vi "joystick control bjorn.vi"() -> ()   [LabVIEW 2016, in "Aerotech VIs.lvlib"]
uses:
  Aerotech VIs.lvlib
  Motion/EnableMultiple.vi
  Motion/HomeSingle.vi
  Motion/DisableMultiple.vi
panel:
  out "Position Feedback":dbl
  in  "u home":bool
  in  "z home":bool
  in  "y home":bool
  in  "x home":bool
  out "U - Position":string
  out "Z - Position":string
  out "Y - Position":string
  out "Selection Number":u32
  in  "U control":bool
  out "u on":bool
  in  "stop":bool
  in  "Joystick On":bool
  in  "Z control":bool
  in  "Y control":bool
  in  "X control":bool
  out "z on":bool
  out "y on":bool
  out "x on":bool
  out "taskId":i32(ring) items=["TLibrary", "T01", "T02", "T03", "T04", "T05", "T06", "T07", "T08", "T09", "T10", "T11", "T12", "T13", "T14", "T15", "T16", "T17", "T18", "T19", "T20", "T21", "T22", "T23", "T24", "T25", "T26", "T27", "T28", "T29", "T30", "T31"]
  # "Do not select more than two values."
  # "Must turn off joystick before changing values. To do so press button on analog stick."
  # "Selection number\nfor establishing\ncase structure value"
  # "X"
  # "Selection number guide:\n#       x-axis       y-axis\n1       NONE         X\n2           Y          NONE\n3           Y              X\n4       NONE         Z\n5           Z              X\n6           Y              Z\n8           U          NONE\n9           U              X\n10         Y              U\n12         U              Z\n\nAll others give no motion"
  # "Y"
  # "Z"
  # "U"
  # "Note:\nX, Y, Z and U are what the various axis are labeled on the gantry. x & y axis refer to the direction on the joypad \nx-axis is left & right\ny-axis is up & down"
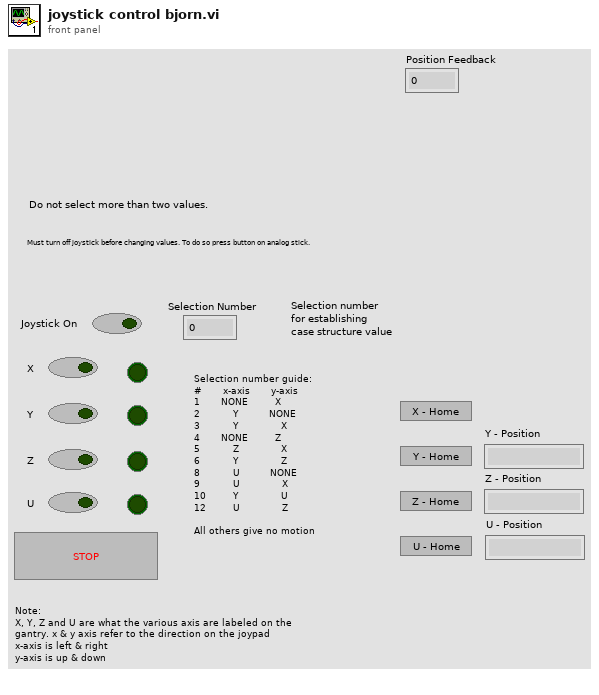
[diagram p1: front panel]
types:
  T1 = typedef "Aerotech VIs.lvlib/ControllerDiagPacket.ctl" = cluster{"Number of Diag Packets":i32, "Axes":T2[], "error":errorcluster}
  T2 = typedef "Aerotech VIs.lvlib/AxisDiagPacket.ctl" = cluster{"Axis Name":string, "Analog Input 0":dbl, "Analog Input 1":dbl, "Axis Fault (num)":i32, "Axis Fault (str)":string, "Axis Fault (bits)":cluster{"AmplifierFault":bool, "AmplifierTemperatureFault":bool, "CcwEndOfTravelLimitFault":bool, "CcwSoftwareLimitFault":bool, "CommunicationLostFault":bool, "CwEndOfTravelLimitFault":bool, "CwSoftwareLimitFault":bool, "EmergencyStopFault":bool, "EncoderFault":bool, "ExternalFault":bool, "FeedbackScalingFault":bool, "GantryMisalignFault ":bool, "HallSensorFault":bool, "InPositionTimeoutFault":bool, "MarkerSearchFault":bool, "MaxVelocityCommandFault":bool, "MotorTemperatureFault":bool, "None":bool, "OverCurrentFault":bool, "PositionErrorFault":bool, "PositionFeedbackFault":bool, "PowerSupplyFault":bool, "ProbeInputFault":bool, "SafeZoneFault":bool, "VelocityErrorFault":bool, "VelocityFeedbackFault":bool, "VoltageClampFault":bool}, "Axis Status (num)":i32, "Axis Status (str)":string, "Axis Status (bits)":cluster{"BacklashActive":bool, "CalibrationEnabled1D":bool, "CalibrationEnabled2D":bool, "CommandValid":bool, "DriveAbortPending":bool, "DrivePending":bool, "Enabling":bool, "GainMappingEnabled":bool, "GantryAligned":bool, "GantryRealigning":bool, "Homed":bool, "Homing":bool, "IFOVEnabled":bool, "JogGenerating":bool, "Jogging":bool, "JoystickControl":bool, "MasterSlaveControl":bool, "MotionBlocked":bool, "MotionClamped":bool, "MoveDone":bool, "None":bool, "NotVirtual":bool, "Profiling":bool, "Stability0":bool, "Stability1":bool, "TrajectoryFiltering":bool, "WaitDone":bool}, "Current Command":sgl, "Current Error":sgl, "Current Feedback":sgl, "Digital Inputs":i32, "Digital Outputs":i32, "Drive Status":i32, "Drive Status (str)":string, "Drive Status (bits)":cluster{"AccelerationPhase":bool, "AutofocusActive":bool, "BrakeOutput":bool, "CcwEndOfTravelLimitInput":bool, "CosineEncoderError":bool, "CurrentClamp":bool, "CwEndOfTravelLimitInput":bool, "DecelerationPhase":bool, "DualLoopActive":bool, "EmergencyStopInput":bool, "Enabled":bool, "EncoderClipping":bool, "GalvoCalibrationEnabled":bool, "GalvoPowerCorrection":bool, "HallAInput":bool, "HallBInput":bool, "HallCInput":bool, "HighResolutionMode":bool, "HomeLimitInput":bool, "InPosition":bool, "InPosition2":bool, "MarkerInput":bool, "MarkerLatch":bool, "MoveActive":bool, "NoMotorSupply":bool, "None":bool, "PowerLimiting":bool, "ProgrammingFlash":bool, "ProgrammingMXH":bool, "PSOHaltLatch":bool, "ServoControl":bool, "SineEncoderError":bool}, "Position Feedback Auxiliary":dbl, "Position Command":dbl, "Position Error":dbl, "Position Feedback":dbl, "Program Position Command":dbl, "Program Position Error":dbl, "Program Position Feedback":dbl, "Velocity Command":dbl, "Velocity Error":dbl, "Velocity Feedback":dbl}
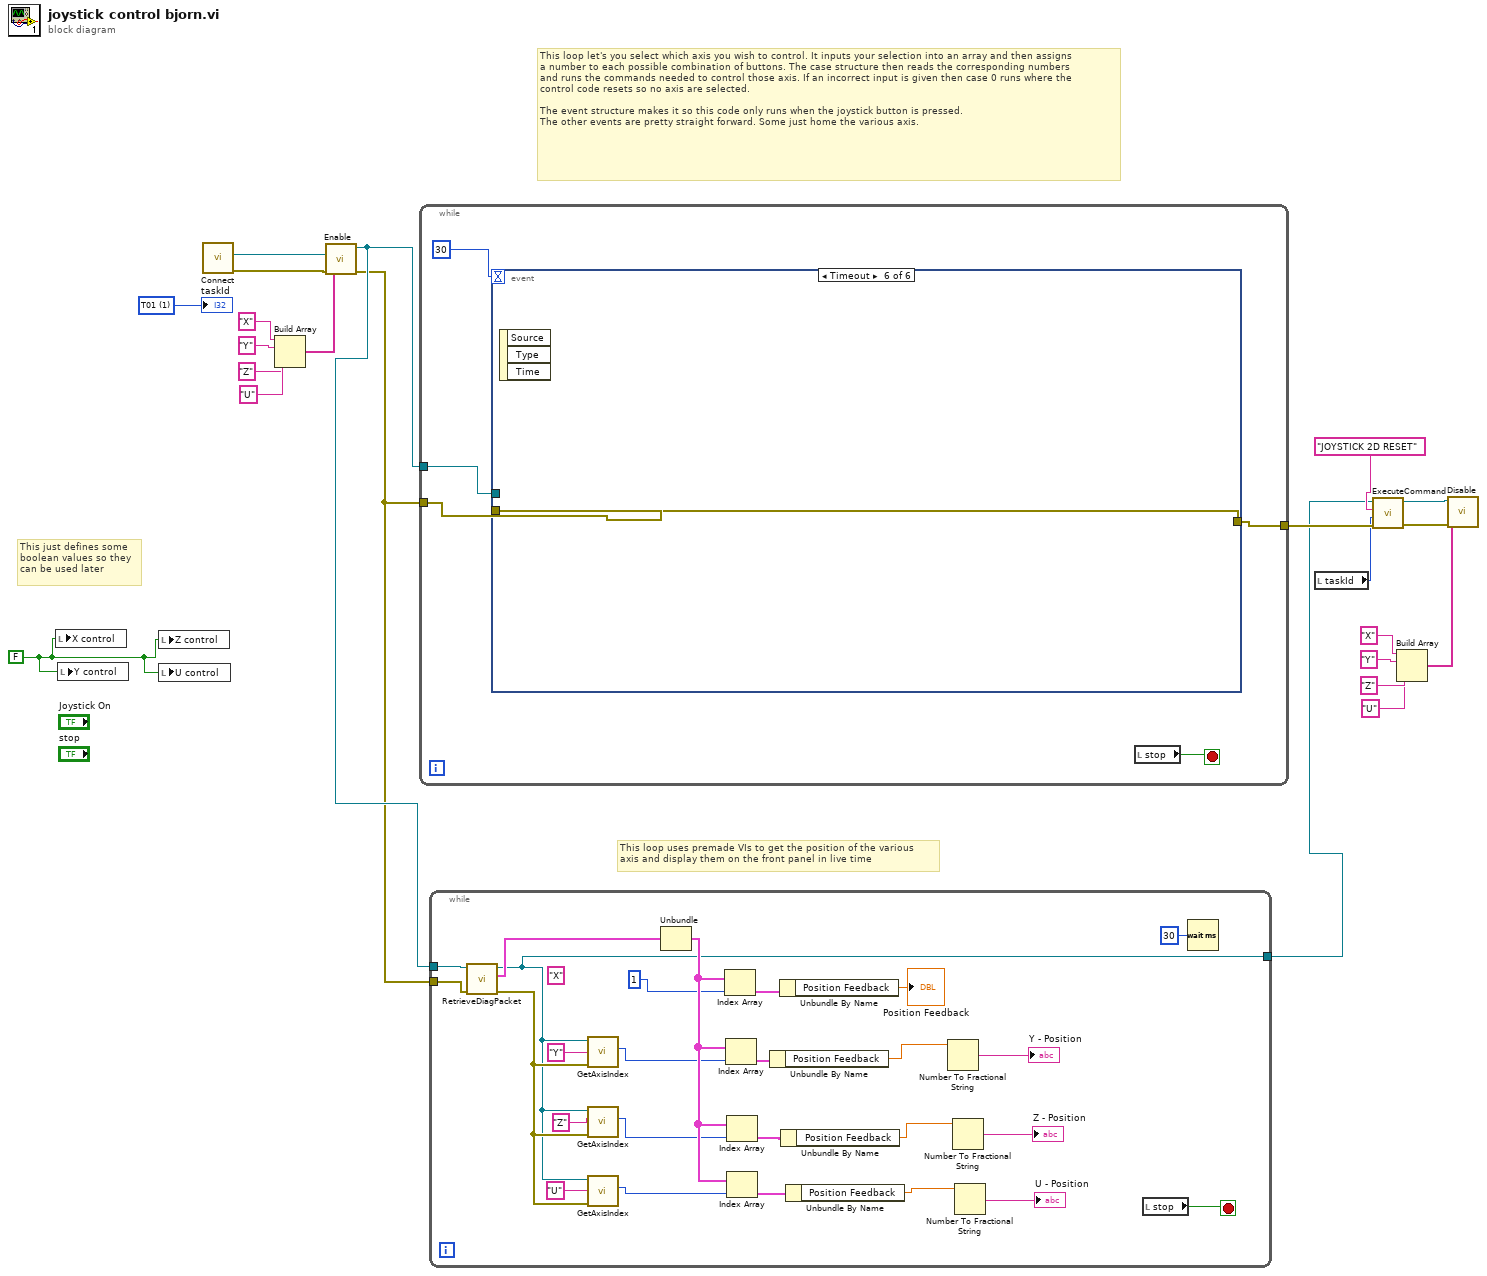
[diagram p0: block diagram]
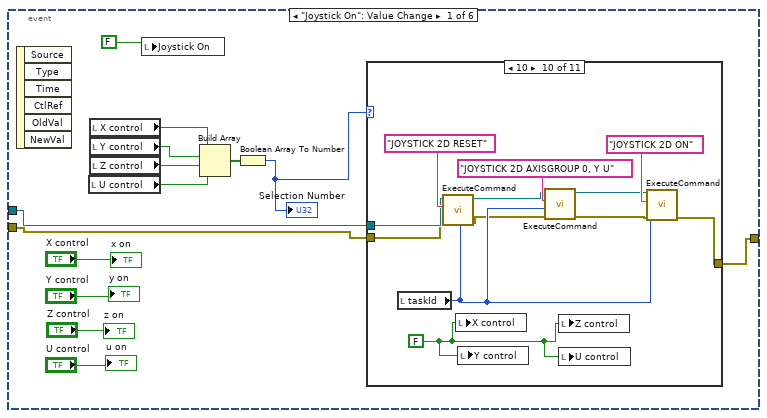
[diagram p2: hidden frame]
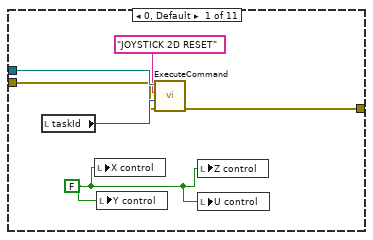
[diagram p3: hidden frame]
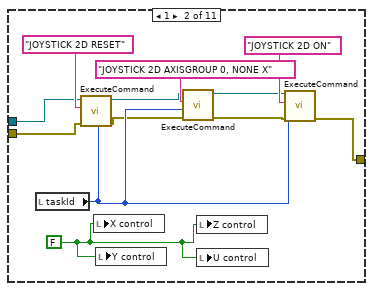
[diagram p4: hidden frame]
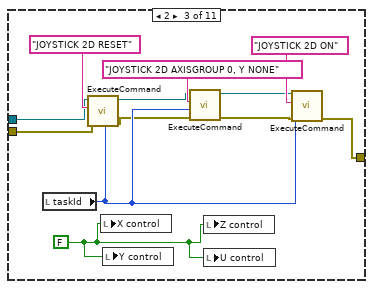
[diagram p5: hidden frame]
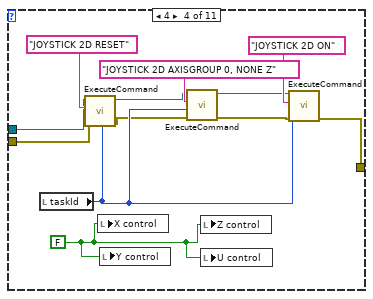
[diagram p6: hidden frame]
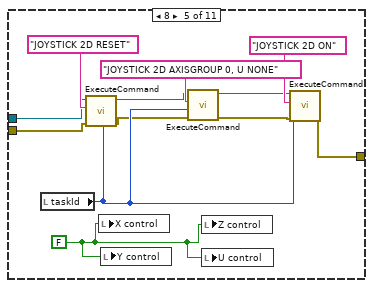
[diagram p7: hidden frame]
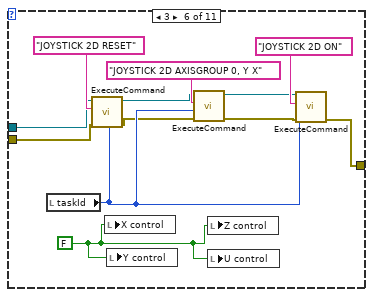
[diagram p8: hidden frame]
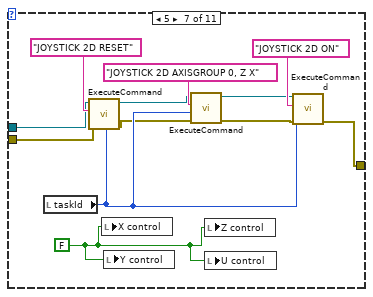
[diagram p9: hidden frame]
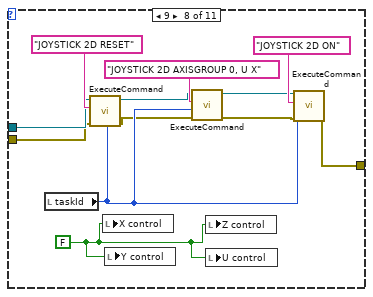
[diagram p10: hidden frame]
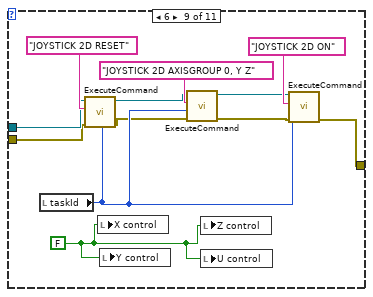
[diagram p11: hidden frame]
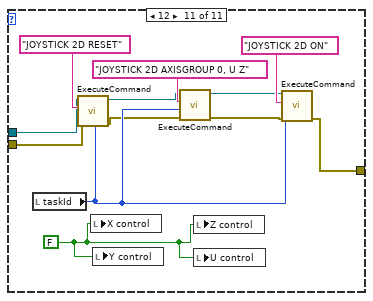
[diagram p12: hidden frame]
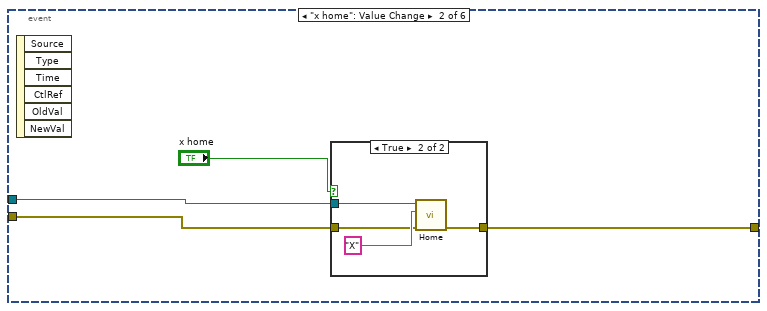
[diagram p13: hidden frame]
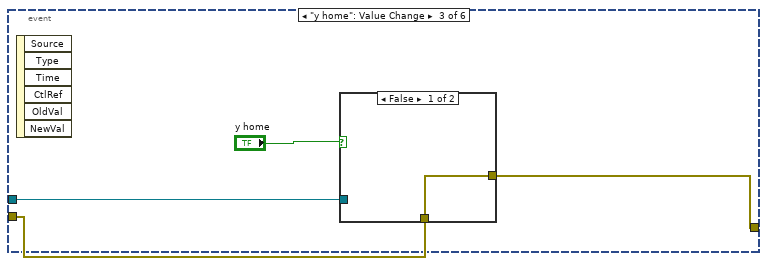
[diagram p15: hidden frame]
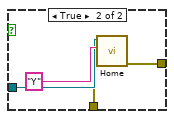
[diagram p16: hidden frame]
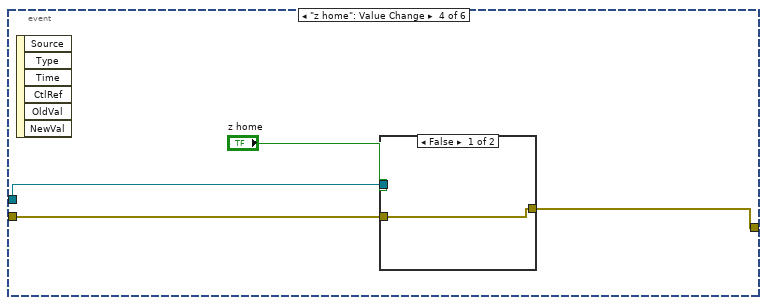
[diagram p17: hidden frame]
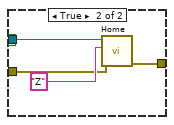
[diagram p18: hidden frame]
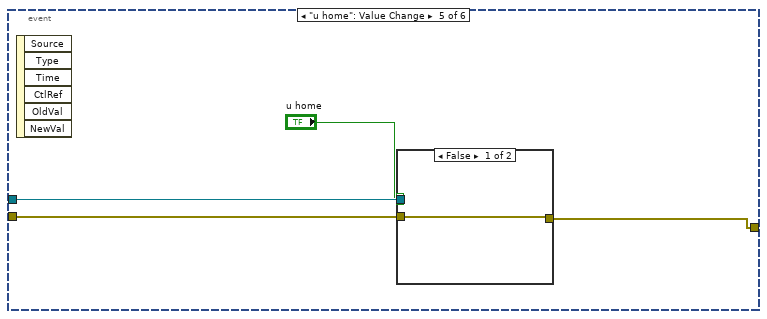
[diagram p19: hidden frame]
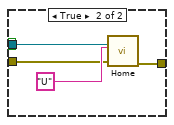
[diagram p20: hidden frame]
diagram:
  w1 = 1 items=["TLibrary", "T01", "T02", "T03", "T04", "T05", "T06", "T07", "T08", "T09", "T10", "T11", "T12", "T13", "T14", "T15", "T16", "T17", "T18", "T19", "T20", "T21", "T22", "T23", "T24", "T25", "T26", "T27", "T28", "T29", "T30", "T31"] ("taskId 2")
  w17 = FALSE
  # "This just defines some\nboolean values so they\ncan be used later"
  # "This loop uses premade VIs to get the position of the various\naxis and display them on the front panel in live time"
  # "This loop let's you select which axis you wish to control. It inputs your selection into an array and then assigns\na number to each possible combination of buttons. The case structure then reads the corresponding numbers\nand runs the commands needed to control those axis. If an incorrect input is given then case 0 runs where the \ncontrol code resets so no axis are selected.\n\nThe event structure makes it so this code only runs when the joystick button is pressed.\nThe other events are pretty straight forward. Some just home the various axis."
  n1 = local write "X control"(w17) -> ()
  n2 = local write "Y control"(w17) -> ()
  n3 = local write "Z control"(w17) -> ()
  n4 = local write "U control"(w17) -> ()
  n5 = call "Connect.vi"() -> ("error out"=w15:errorcluster, "controller"=w16:refnum<k24>)  [unwired: 10 in]
  n6 = Build Array("X", "Y", "Z", "U") -> (w18:string[])
  n7 = call-poly "Enable.vi"("error in (no error)"=w15, "axis names"=w18, "controller in"=w16) -> ("error out"=w13:errorcluster, "controller out"=w14:refnum<k24>)  [unwired: 7 in]
  n8 = while {
    tunnel: w14 -> [w24]
    tunnel: w13 -> [w26]
    tunnel: [w23] -> w11
    stop <- w25 stop-if-true
    n9 = event shown="[5] Timeout" {
      selector: _ -> [_ _ _ _ _ _]
      dyn-events: _ -> [_ _ _ _ _ _]
      timeout: 30 -> [_ _ _ _ _ _]
      tunnel: w26 -> [w30 w170 w179 w188 w197 w204]
      tunnel: w24 -> [w31 w171 w180 w189 w198 _]
      tunnel: [w28 w168 w177 w186 w195 w204] -> w23
      event "Joystick On": Value Change {
        n10 = event-data() -> ()  [unwired: 1 in, 6 out]
        n11 = local read "U control"() -> (w38:bool)
        n12 = local read "X control"() -> (w41:bool)
        n13 = local read "Y control"() -> (w40:bool)
        n14 = local read "Z control"() -> (w39:bool)
        n15 = local write "Joystick On"(FALSE) -> ()
        n16 = Build Array(w41, w40, w39, w38) -> (w37:bool[])
        n17 = Boolean Array To Number(Boolean array=w37) -> (number=w36:u32)
        "Selection Number" <- w36
        n18 = case shown="10" w36 {
          tunnel: w31 -> [w45 w51 w62 w73 w86 w98 w110 w122 w134 w146 w158]
          tunnel: w30 -> [w44 w50 w61 w74 w85 w97 w109 w121 w133 w145 w157]
          tunnel: [w42 w48 w60 w72 w84 w96 w108 w120 w132 w144 w156] -> w28
          frame 0, Default {
            w47 = FALSE
            n19 = local read "taskId"() -> (w46:i32)
            n20 = local write "X control"(w47) -> ()
            n21 = local write "Y control"(w47) -> ()
            n22 = call "ExecuteCommand.vi"("error in (no error)"=w44, "taskId"=w46, "Command Code"="JOYSTICK 2D RESET", "controller in"=w45) -> ("error out"=w42:errorcluster)  [unwired: 5 in, 2 out]
            n23 = local write "Z control"(w47) -> ()
            n24 = local write "U control"(w47) -> ()
          }
          frame 1 {
            w49 = FALSE
            n25 = local read "taskId"() -> (w56:i32)
            n26 = call "ExecuteCommand.vi"("error in (no error)"=w50, "taskId"=w56, "Command Code"="JOYSTICK 2D RESET", "controller in"=w51) -> ("error out"=w52:errorcluster, "controller out"=w55:refnum<k24>)  [unwired: 5 in, 1 out]
            n27 = local write "X control"(w49) -> ()
            n28 = local write "Y control"(w49) -> ()
            n29 = call "ExecuteCommand.vi"("error in (no error)"=w52, "taskId"=w56, "Command Code"="JOYSTICK 2D AXISGROUP 0, NONE X", "controller in"=w55) -> ("error out"=w53:errorcluster, "controller out"=w54:refnum<k24>)  [unwired: 5 in, 1 out]
            n30 = local write "Z control"(w49) -> ()
            n31 = local write "U control"(w49) -> ()
            n32 = call "ExecuteCommand.vi"("error in (no error)"=w53, "taskId"=w56, "Command Code"="JOYSTICK 2D ON", "controller in"=w54) -> ("error out"=w48:errorcluster)  [unwired: 5 in, 2 out]
          }
          frame 2 {
            w63 = FALSE
            n33 = local read "taskId"() -> (w68:i32)
            n34 = call "ExecuteCommand.vi"("error in (no error)"=w61, "taskId"=w68, "Command Code"="JOYSTICK 2D RESET", "controller in"=w62) -> ("error out"=w64:errorcluster, "controller out"=w67:refnum<k24>)  [unwired: 5 in, 1 out]
            n35 = local write "X control"(w63) -> ()
            n36 = local write "Y control"(w63) -> ()
            n37 = call "ExecuteCommand.vi"("error in (no error)"=w64, "taskId"=w68, "Command Code"="JOYSTICK 2D AXISGROUP 0, Y NONE", "controller in"=w67) -> ("error out"=w65:errorcluster, "controller out"=w66:refnum<k24>)  [unwired: 5 in, 1 out]
            n38 = local write "Z control"(w63) -> ()
            n39 = local write "U control"(w63) -> ()
            n40 = call "ExecuteCommand.vi"("error in (no error)"=w65, "taskId"=w68, "Command Code"="JOYSTICK 2D ON", "controller in"=w66) -> ("error out"=w60:errorcluster)  [unwired: 5 in, 2 out]
          }
          frame 4 {
            w75 = FALSE
            n41 = local read "taskId"() -> (w80:i32)
            n42 = call "ExecuteCommand.vi"("error in (no error)"=w74, "taskId"=w80, "Command Code"="JOYSTICK 2D RESET", "controller in"=w73) -> ("error out"=w76:errorcluster, "controller out"=w79:refnum<k24>)  [unwired: 5 in, 1 out]
            n43 = local write "X control"(w75) -> ()
            n44 = local write "Y control"(w75) -> ()
            n45 = call "ExecuteCommand.vi"("error in (no error)"=w76, "taskId"=w80, "Command Code"="JOYSTICK 2D AXISGROUP 0, NONE Z", "controller in"=w79) -> ("error out"=w77:errorcluster, "controller out"=w78:refnum<k24>)  [unwired: 5 in, 1 out]
            n46 = local write "Z control"(w75) -> ()
            n47 = local write "U control"(w75) -> ()
            n48 = call "ExecuteCommand.vi"("error in (no error)"=w77, "taskId"=w80, "Command Code"="JOYSTICK 2D ON", "controller in"=w78) -> ("error out"=w72:errorcluster)  [unwired: 5 in, 2 out]
          }
          frame 8 {
            w87 = FALSE
            n49 = local read "taskId"() -> (w92:i32)
            n50 = call "ExecuteCommand.vi"("error in (no error)"=w85, "taskId"=w92, "Command Code"="JOYSTICK 2D RESET", "controller in"=w86) -> ("error out"=w88:errorcluster, "controller out"=w91:refnum<k24>)  [unwired: 5 in, 1 out]
            n51 = local write "X control"(w87) -> ()
            n52 = local write "Y control"(w87) -> ()
            n53 = call "ExecuteCommand.vi"("error in (no error)"=w88, "taskId"=w92, "Command Code"="JOYSTICK 2D AXISGROUP 0, U NONE", "controller in"=w91) -> ("error out"=w89:errorcluster, "controller out"=w90:refnum<k24>)  [unwired: 5 in, 1 out]
            n54 = local write "Z control"(w87) -> ()
            n55 = local write "U control"(w87) -> ()
            n56 = call "ExecuteCommand.vi"("error in (no error)"=w89, "taskId"=w92, "Command Code"="JOYSTICK 2D ON", "controller in"=w90) -> ("error out"=w84:errorcluster)  [unwired: 5 in, 2 out]
          }
          frame 3 {
            w99 = FALSE
            n57 = local read "taskId"() -> (w104:i32)
            n58 = call "ExecuteCommand.vi"("error in (no error)"=w97, "taskId"=w104, "Command Code"="JOYSTICK 2D RESET", "controller in"=w98) -> ("error out"=w100:errorcluster, "controller out"=w103:refnum<k24>)  [unwired: 5 in, 1 out]
            n59 = local write "X control"(w99) -> ()
            n60 = local write "Y control"(w99) -> ()
            n61 = call "ExecuteCommand.vi"("error in (no error)"=w100, "taskId"=w104, "Command Code"="JOYSTICK 2D AXISGROUP 0, Y X", "controller in"=w103) -> ("error out"=w101:errorcluster, "controller out"=w102:refnum<k24>)  [unwired: 5 in, 1 out]
            n62 = local write "Z control"(w99) -> ()
            n63 = local write "U control"(w99) -> ()
            n64 = call "ExecuteCommand.vi"("error in (no error)"=w101, "taskId"=w104, "Command Code"="JOYSTICK 2D ON", "controller in"=w102) -> ("error out"=w96:errorcluster)  [unwired: 5 in, 2 out]
          }
          frame 5 {
            w111 = FALSE
            n65 = local read "taskId"() -> (w116:i32)
            n66 = call "ExecuteCommand.vi"("error in (no error)"=w109, "taskId"=w116, "Command Code"="JOYSTICK 2D RESET", "controller in"=w110) -> ("error out"=w112:errorcluster, "controller out"=w115:refnum<k24>)  [unwired: 5 in, 1 out]
            n67 = local write "X control"(w111) -> ()
            n68 = local write "Y control"(w111) -> ()
            n69 = call "ExecuteCommand.vi"("error in (no error)"=w112, "taskId"=w116, "Command Code"="JOYSTICK 2D AXISGROUP 0, Z X", "controller in"=w115) -> ("error out"=w113:errorcluster, "controller out"=w114:refnum<k24>)  [unwired: 5 in, 1 out]
            n70 = local write "Z control"(w111) -> ()
            n71 = local write "U control"(w111) -> ()
            n72 = call "ExecuteCommand.vi"("error in (no error)"=w113, "taskId"=w116, "Command Code"="JOYSTICK 2D ON", "controller in"=w114) -> ("error out"=w108:errorcluster)  [unwired: 5 in, 2 out]
          }
          frame 9 {
            w123 = FALSE
            n73 = local read "taskId"() -> (w128:i32)
            n74 = call "ExecuteCommand.vi"("error in (no error)"=w121, "taskId"=w128, "Command Code"="JOYSTICK 2D RESET", "controller in"=w122) -> ("error out"=w124:errorcluster, "controller out"=w127:refnum<k24>)  [unwired: 5 in, 1 out]
            n75 = local write "X control"(w123) -> ()
            n76 = local write "Y control"(w123) -> ()
            n77 = call "ExecuteCommand.vi"("error in (no error)"=w124, "taskId"=w128, "Command Code"="JOYSTICK 2D AXISGROUP 0, U X", "controller in"=w127) -> ("error out"=w125:errorcluster, "controller out"=w126:refnum<k24>)  [unwired: 5 in, 1 out]
            n78 = local write "Z control"(w123) -> ()
            n79 = local write "U control"(w123) -> ()
            n80 = call "ExecuteCommand.vi"("error in (no error)"=w125, "taskId"=w128, "Command Code"="JOYSTICK 2D ON", "controller in"=w126) -> ("error out"=w120:errorcluster)  [unwired: 5 in, 2 out]
          }
          frame 6 {
            w135 = FALSE
            n81 = local read "taskId"() -> (w140:i32)
            n82 = call "ExecuteCommand.vi"("error in (no error)"=w133, "taskId"=w140, "Command Code"="JOYSTICK 2D RESET", "controller in"=w134) -> ("error out"=w136:errorcluster, "controller out"=w139:refnum<k24>)  [unwired: 5 in, 1 out]
            n83 = local write "X control"(w135) -> ()
            n84 = local write "Y control"(w135) -> ()
            n85 = call "ExecuteCommand.vi"("error in (no error)"=w136, "taskId"=w140, "Command Code"="JOYSTICK 2D AXISGROUP 0, Y Z", "controller in"=w139) -> ("error out"=w137:errorcluster, "controller out"=w138:refnum<k24>)  [unwired: 5 in, 1 out]
            n86 = local write "Z control"(w135) -> ()
            n87 = local write "U control"(w135) -> ()
            n88 = call "ExecuteCommand.vi"("error in (no error)"=w137, "taskId"=w140, "Command Code"="JOYSTICK 2D ON", "controller in"=w138) -> ("error out"=w132:errorcluster)  [unwired: 5 in, 2 out]
          }
          frame 10 {
            w147 = FALSE
            n89 = local read "taskId"() -> (w152:i32)
            n90 = call "ExecuteCommand.vi"("error in (no error)"=w145, "taskId"=w152, "Command Code"="JOYSTICK 2D RESET", "controller in"=w146) -> ("error out"=w148:errorcluster, "controller out"=w151:refnum<k24>)  [unwired: 5 in, 1 out]
            n91 = local write "X control"(w147) -> ()
            n92 = local write "Y control"(w147) -> ()
            n93 = call "ExecuteCommand.vi"("error in (no error)"=w148, "taskId"=w152, "Command Code"="JOYSTICK 2D AXISGROUP 0, Y U", "controller in"=w151) -> ("error out"=w149:errorcluster, "controller out"=w150:refnum<k24>)  [unwired: 5 in, 1 out]
            n94 = local write "Z control"(w147) -> ()
            n95 = local write "U control"(w147) -> ()
            n96 = call "ExecuteCommand.vi"("error in (no error)"=w149, "taskId"=w152, "Command Code"="JOYSTICK 2D ON", "controller in"=w150) -> ("error out"=w144:errorcluster)  [unwired: 5 in, 2 out]
          }
          frame 12 {
            w159 = FALSE
            n97 = local read "taskId"() -> (w164:i32)
            n98 = call "ExecuteCommand.vi"("error in (no error)"=w157, "taskId"=w164, "Command Code"="JOYSTICK 2D RESET", "controller in"=w158) -> ("error out"=w160:errorcluster, "controller out"=w163:refnum<k24>)  [unwired: 5 in, 1 out]
            n99 = local write "X control"(w159) -> ()
            n100 = local write "Y control"(w159) -> ()
            n101 = call "ExecuteCommand.vi"("error in (no error)"=w160, "taskId"=w164, "Command Code"="JOYSTICK 2D AXISGROUP 0, U Z", "controller in"=w163) -> ("error out"=w161:errorcluster, "controller out"=w162:refnum<k24>)  [unwired: 5 in, 1 out]
            n102 = local write "Z control"(w159) -> ()
            n103 = local write "U control"(w159) -> ()
            n104 = call "ExecuteCommand.vi"("error in (no error)"=w161, "taskId"=w164, "Command Code"="JOYSTICK 2D ON", "controller in"=w162) -> ("error out"=w156:errorcluster)  [unwired: 5 in, 2 out]
          }
        }
        "x on" <- "X control"
        "y on" <- "Y control"
        "z on" <- "Z control"
        "u on" <- "U control"
      }
      event "x home": Value Change {
        n105 = event-data() -> ()  [unwired: 1 in, 6 out]
        n106 = case shown="True" "x home" {
          tunnel: w171 -> [_ w175]
          tunnel: w170 -> [w172 w174]
          tunnel: [w172 w173] -> w168
          frame False {
          }
          frame True {
            n107 = call-poly "Home.vi"("error in (no error)"=w174, "axis name"="X", "controller in"=w175) -> ("error out"=w173:errorcluster)  [unwired: 7 in, 1 out]
          }
        }
      }
      event "y home": Value Change {
        n108 = event-data() -> ()  [unwired: 1 in, 6 out]
        n109 = case shown="False" "y home" {
          tunnel: w180 -> [_ w184]
          tunnel: w179 -> [w181 w183]
          tunnel: [w181 w182] -> w177
          frame False {
          }
          frame True {
            n110 = call-poly "Home.vi"("error in (no error)"=w183, "axis name"="Y", "controller in"=w184) -> ("error out"=w182:errorcluster)  [unwired: 7 in, 1 out]
          }
        }
      }
      event "z home": Value Change {
        n111 = event-data() -> ()  [unwired: 1 in, 6 out]
        n112 = case shown="False" "z home" {
          tunnel: w189 -> [_ w193]
          tunnel: w188 -> [w190 w192]
          tunnel: [w190 w191] -> w186
          frame False {
          }
          frame True {
            n113 = call-poly "Home.vi"("error in (no error)"=w192, "axis name"="Z", "controller in"=w193) -> ("error out"=w191:errorcluster)  [unwired: 7 in, 1 out]
          }
        }
      }
      event "u home": Value Change {
        n114 = event-data() -> ()  [unwired: 1 in, 6 out]
        n115 = case shown="False" "u home" {
          tunnel: w198 -> [_ w202]
          tunnel: w197 -> [w199 w201]
          tunnel: [w199 w200] -> w195
          frame False {
          }
          frame True {
            n116 = call-poly "Home.vi"("error in (no error)"=w201, "axis name"="U", "controller in"=w202) -> ("error out"=w200:errorcluster)  [unwired: 7 in, 1 out]
          }
        }
      }
      event Timeout {
        n117 = event-data() -> ()  [unwired: 1 in, 3 out]
      }
    }
    n118 = local read "stop"() -> (w25:bool)
  }
  n119 = while {
    tunnel: w14 -> [w224]
    tunnel: w13 -> [w223]
    tunnel: [w209] -> w2
    stop <- w210 stop-if-true
    (unwired) "X"
    n120 = call "RetrieveDiagPacket.vi"("error in (no error)"=w223, "Controller In"=w224) -> ("error out"=w227:errorcluster, "ControllerDiagPacket"=w226:T1, "Controller Out"=w209:refnum<k24>)  [unwired: 7 in]
    n121 = call "GetAxisIndex.vi"("error in (no error)"=w227, "axis name"="Y", "controller in"=w209) -> ("axis index"=w221:i32)  [unwired: 6 in, 2 out]
    n122 = call "GetAxisIndex.vi"("error in (no error)"=w227, "axis name"="Z", "controller in"=w209) -> ("axis index"=w220:i32)  [unwired: 6 in, 2 out]
    n123 = call "GetAxisIndex.vi"("error in (no error)"=w227, "axis name"="U", "controller in"=w209) -> ("axis index"=w219:i32)  [unwired: 6 in, 2 out]
    n124 = Unbundle(w226) -> ("Axes"=w225:T2[])  [unwired: 2 out]
    n125 = Index Array(array=w225, index=1) -> (element=w218:T2)
    n126 = Index Array(array=w225, index=w221) -> (element=w216:T2)
    n127 = Index Array(array=w225, index=w220) -> (element=w215:T2)
    n128 = Index Array(array=w225, index=w219) -> (element=w217:T2)
    n129 = Unbundle By Name(w216) -> ("Position Feedback"=w208:dbl)
    n130 = Unbundle By Name(w218) -> ("Position Feedback"=→"Position Feedback":dbl)
    n131 = Unbundle By Name(w215) -> ("Position Feedback"=w214:dbl)
    n132 = Unbundle By Name(w217) -> ("Position Feedback"=w207:dbl)
    n133 = Number To Fractional String(number=w208) -> (F-format string=→"Y - Position":string)  [unwired: 3 in]
    n134 = Number To Fractional String(number=w214) -> (F-format string=→"Z - Position":string)  [unwired: 3 in]
    n135 = Number To Fractional String(number=w207) -> (F-format string=→"U - Position":string)  [unwired: 3 in]
    n136 = local read "stop"() -> (w210:bool)
    n137 = Wait (ms)(milliseconds to wait=u32 30) -> ()  [unwired: 1 out]
  }
  n138 = local read "taskId"() -> (w10:i32)
  n139 = call "ExecuteCommand.vi"("error in (no error)"=w11, "taskId"=w10, "Command Code"="JOYSTICK 2D RESET", "controller in"=w2) -> ("error out"=w8:errorcluster, "controller out"=w9:refnum<k24>)  [unwired: 5 in, 1 out]
  n140 = Build Array("X", "Y", "Z", "U") -> (w3:string[])
  n141 = call-poly "Disable.vi"("error in (no error)"=w8, "axis names"=w3, "controller in"=w9) -> ()  [unwired: 7 in, 2 out]
  "taskId" <- w1
